vi "NewCreatorB.vi"(8 "error in (no error)":errorcluster) -> (0 "error out":errorcluster, 3 "CreatorB":refnum<class "CreatorB.lvclass">)   [LabVIEW 2020, in "FactoryMethod.lvlib" / "FactoryMethodLazyEvaluation.lvlib" / "CreatorB.lvclass"]
uses:
  CreatorB.lvclass
  CreatorB.lvclass/CreatorB.ctl
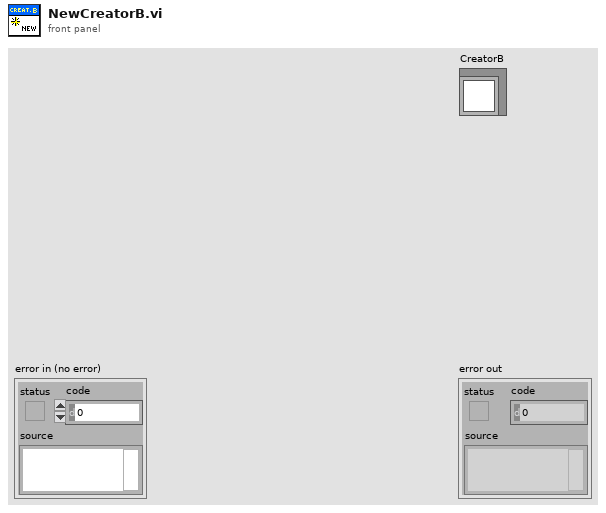
[diagram p1: front panel]
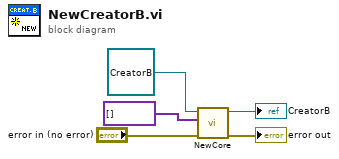
[diagram p0: block diagram]
diagram:
  n1 = call-dynamic "NewCore.vi"("error in (no error)"="error in (no error)", "ParamsArray"=variant[] [], "CreatorB"=refnum<class "CreatorB.lvclass"> refnum ("ConcreteCreatorA in")) -> ("error out"=→"error out":errorcluster, "CreatorB"=→"CreatorB":refnum<class "CreatorB.lvclass">)  [unwired: 7 in]
